vi "QCA Current to Channel Array.vi"(0 "Channel Number":i32) -> ()   [LabVIEW 2009]
doc: "This VI takes channel info from the QCA Global and shuffles it back into the Channel Array. It's easier to do it this way than the alternative, which would be to de-index the correct element of the channel array each time a setting in the channel is changed."
uses:
  QCA Global.vi
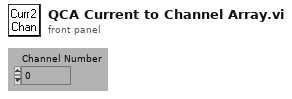
[diagram p1: front panel]
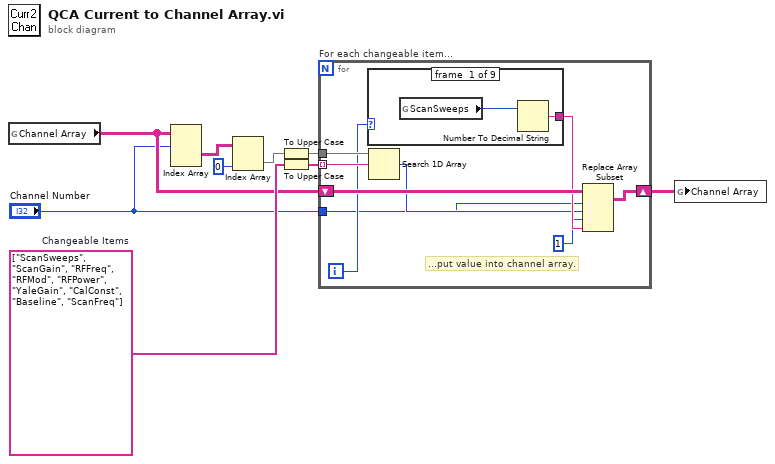
[diagram p0: block diagram]
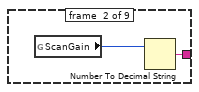
[diagram p2: hidden frame]
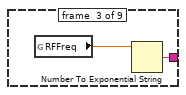
[diagram p3: hidden frame]
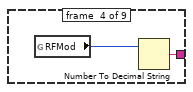
[diagram p4: hidden frame]
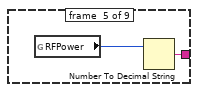
[diagram p5: hidden frame]
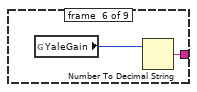
[diagram p6: hidden frame]
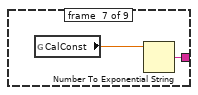
[diagram p7: hidden frame]
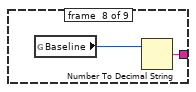
[diagram p8: hidden frame]
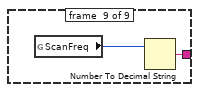
[diagram p9: hidden frame]
diagram:
  w7 = string[] ["ScanSweeps", "ScanGain", "RFFreq", "RFMod", "RFPower", "YaleGain", "CalConst", "Baseline", "ScanFreq"]  # Changeable Items
  n1 = global read "QCA Global.vi" "Channel Array"() -> (w4:string[][][])
  n2 = Index Array(array=w4, index (dim 0)="Channel Number") -> (element=w9:string[][])  [unwired: 2 in]
  n3 = Index Array(array=w9, index (col)=0 ("Index")) -> (element=w3:string[])  [unwired: 1 in]
  n4 = To Upper Case(1:w3) -> (0:w6:string[])
  n5 = To Upper Case(1:w7) -> (0:w5:string[])
  n6 = for "For each changeable item..." {
    tunnel: w6 -> [w18]
    shift-right: [w16] -> w2
    shift-left: w4 -> [w17]
    tunnel: w5 -> [w15] mode=indexing
    tunnel: "Channel Number" -> [w11]
    i -> [w13]
    # "...put value into channel array."
    n7 = case shown="8" w13 {
      tunnel: [w19 w21 w23 w25 w27 w29 w31 w33 w35] -> w14
      frame #0 {
        n8 = global read "QCA Global.vi" "ScanSweeps"() -> (w20:i32)
        n9 = Number To Decimal String(number=w20) -> (decimal integer string=w19:string)  [unwired: 1 in]
      }
      frame #1 {
        n10 = global read "QCA Global.vi" "ScanGain"() -> (w22:i32)
        n11 = Number To Decimal String(number=w22) -> (decimal integer string=w21:string)  [unwired: 1 in]
      }
      frame #2 {
        n12 = global read "QCA Global.vi" "RFFreq"() -> (w24:dbl)
        n13 = Number To Exponential String(number=w24) -> (E-format string=w23:string)  [unwired: 3 in]
      }
      frame #3 {
        n14 = global read "QCA Global.vi" "RFMod"() -> (w26:i32)
        n15 = Number To Decimal String(number=w26) -> (decimal integer string=w25:string)  [unwired: 1 in]
      }
      frame #4 {
        n16 = global read "QCA Global.vi" "RFPower"() -> (w28:i32)
        n17 = Number To Decimal String(number=w28) -> (decimal integer string=w27:string)  [unwired: 1 in]
      }
      frame #5 {
        n18 = global read "QCA Global.vi" "YaleGain"() -> (w30:i32)
        n19 = Number To Decimal String(number=w30) -> (decimal integer string=w29:string)  [unwired: 1 in]
      }
      frame #6 {
        n20 = global read "QCA Global.vi" "CalConst"() -> (w32:dbl)
        n21 = Number To Exponential String(number=w32) -> (E-format string=w31:string)  [unwired: 3 in]
      }
      frame #7 {
        n22 = global read "QCA Global.vi" "Baseline"() -> (w34:i32)
        n23 = Number To Decimal String(number=w34) -> (decimal integer string=w33:string)  [unwired: 1 in]
      }
      frame #8 {
        n24 = global read "QCA Global.vi" "ScanFreq"() -> (w36:i32)
        n25 = Number To Decimal String(number=w36) -> (decimal integer string=w35:string)  [unwired: 1 in]
      }
    }
    n26 = Search 1D Array(1D array=w18, element=w15) -> (index of element=w12:i32)  [unwired: 1 in]
    n27 = Replace Array Subset(array=w17, new element=w14, index (dim 0)=w11, index (dim 1)=w12, index (dim 2)=1 ("Index")) -> (w16:string[][][])
  }
  n28 = global write "QCA Global.vi" "Channel Array"(w2) -> ()
